vi "Field Draw Balls.vi"(3 "Project":T2=enum."VSS", 4 "Draw Targets?":T3, 5 "KeeperPlay":T1=enum."NormalGame", 6 "side":enum16{"Esquerdo", "Direito"}(ring), 7 "Referee":refnum<class "Referee.lvclass">=refnum, 8 "Picture In":picture, 9 "Offset":cluster{"Width":dbl, "Height":dbl}, 10 "Scale":dbl, 11 "BallRef":refnum<class "Ball.lvclass">=refnum) -> (0 "Picture Out":picture, 1 "Offset Out":cluster{"Width":dbl, "Height":dbl}, 2 "Scale Out":dbl)   [LabVIEW 2022 SP3]
uses:
  Ball_class/Ball.lvclass
  DrawTargets.ctl
  Project.ctl
  Referee_class/Referee.lvclass
  Team_class/KeeperPlay.ctl
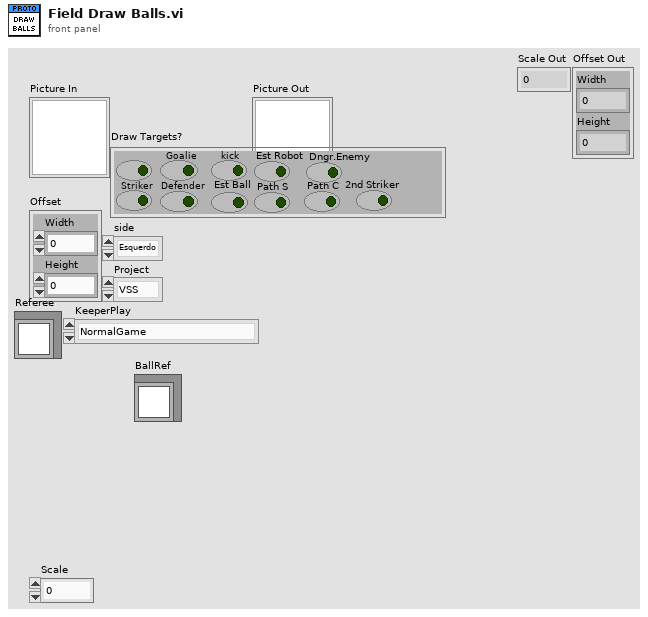
[diagram p1: front panel]
types:
  T1 = typedef "KeeperPlay.ctl" = enum16{"ZigZag", "BallPlacement", "Goto", "NormalGame", "KeeperPlay", "Halt", "Timeout", "PenaltyEnemy", "TestPlay"}
  T2 = typedef "Project.ctl" = enum16{"SSL", "VSS"}
  T3 = typedef "DrawTargets.ctl" = cluster{"Attacker":bool, "Striker":bool, "Goalie":bool, "Defender":bool, "kick":bool, "Est Ball":bool, "Est Robot":bool, "Path S":bool, "Path C":bool, "Dngr.Enemy":bool, "2nd Striker":bool}
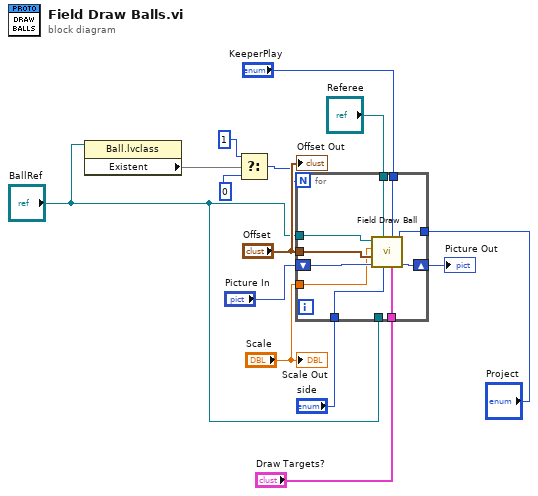
[diagram p0: block diagram]
diagram:
  n1 = property class="Ball.lvclass"(reference="BallRef") -> ("Existent"=w5)  [unwired: 1 in, 2 out]
  n2 = Select(t=1, s=w5, f=0) -> (s? t:f=w7:i32)
  n3 = for {
    N: w7 -> [_]
    tunnel: "Scale" -> [w20]
    tunnel: "Offset" -> [w21]
    tunnel: "BallRef" -> [w22]
    shift-right: [w24] -> w11
    shift-left: "Picture In" -> [w23]
    tunnel: "BallRef" -> [_]
    tunnel: "Draw Targets?" -> [w19]
    tunnel: "side" -> [w18]
    tunnel: "Project" -> [w17]
    tunnel: "Referee" -> [w16]
    tunnel: "KeeperPlay" -> [w15]
    n4 = call "Field Draw Ball.vi"("Project"=w17, "Draw Targets?"=w19, "KeeperPlay"=w15, "Lado"=w18, "Referee"=w16, "picture in"=w23, "Offset"=w21, "Scale mm/pixel"=w20, "BallRef"=w22) -> ("picture out"=w24:picture)  [unwired: 2 in]
  }
  "Picture Out" <- w11
  "Scale Out" <- "Scale"
  "Offset Out" <- "Offset"
